vi "Directory Separator.vi"() -> (0 "Directory Separator":string)   [LabVIEW 2020, in "AoC 2022.lvlib"]
uses:
  AoC 2022.lvlib
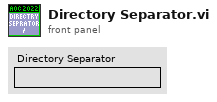
[diagram p1: front panel]
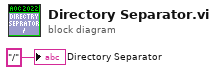
[diagram p0: block diagram]
diagram:
  "Directory Separator" <- "/"
